vi "glob1.vi"() -> ()   [LabVIEW 2010]
uses:
  <instrlib>/niScope/Controls/niScope vertical coupling.ctl
  <instrlib>/niScope/Controls/niScope trigger slope.ctl
  <instrlib>/niScope/Controls/niScope trigger source digital.ctl
panel:
  in  "Tabs":enum32{"Усилитель", "ScopeSettings"}(tab)
  in  "TAI-GPS":dbl=34.0
  in  "Array":dbl[](array[numeric])=[40.0, 20.0, 10.0, 4.0, 2.0, 1.0, 0.4, 0.2, 0.1, 0.04] caption="Диапазон / Шкала"
  in  "DigitalTrigger":T3={"slope"=0, "source"="VAL_RTSI_4", "holdoff"=0.0, "delay"=0.0} {"delay" format="%#.6g"}
  in  "HorizontalTiming":T4={"enforce realtime"=FALSE, "number of records"=1, "min sample rate"=125000000.0, "reference position"=0.0, "min record length"=4000000} {"min sample rate" format="%#_6p"}
  in  "channel parameters":T6(array[cluster])=[{"channel name"="0", "input impedance"=0, "maximum input frequency"=0.0, "vertical coupling"=1, "probe attenuation"=1.0, "vertical range"=2.0, "vertical offset"=0.0, "channel enabled"=TRUE}, {"channel name"="1", "input impedance"=0, "maximum input frequency"=0.0, "vertical coupling"=1, "probe attenuation"=1.0, "vertical range"=2.0, "vertical offset"=0.0, "channel enabled"=TRUE}] {"vertical coupling" items=["AC", "DC", "Ground"]; "input impedance" items=["1 mega ohm"=0, "50 ohms"=2]}
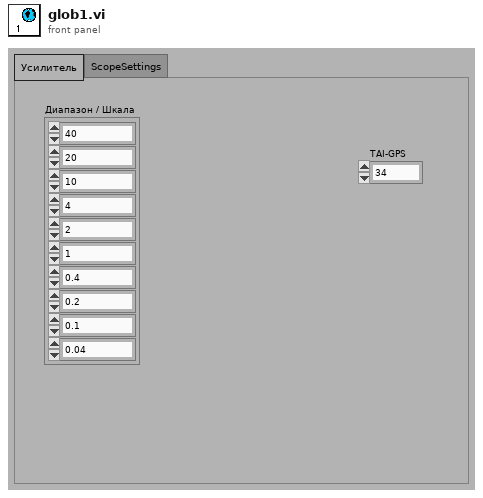
[diagram p1: front panel]
types:
  T1 = typedef "niScope trigger slope.ctl" = i32
  T2 = typedef "niScope trigger source digital.ctl" = string
  T3 = cluster{"slope":T1, "source":T2, "holdoff":dbl, "delay":dbl}
  T4 = cluster{"enforce realtime":bool, "number of records":i32, "min sample rate":dbl, "reference position":dbl, "min record length":i32}
  T5 = typedef "niScope vertical coupling.ctl" = i32
  T6 = cluster{"channel name":string, "input impedance":u32, "maximum input frequency":dbl, "vertical coupling":T5, "probe attenuation":dbl, "vertical range":dbl, "vertical offset":dbl, "channel enabled":bool}[]
diagram:
